vi "L_Cal_Data_Dis_Reflectivity.vi"(9 "Index(0 or 1)":i32, 10 "ID":i32, 11 "data":u8[](array[numeric])) -> (2 "reflectivity":u8, 3 "Distance":dbl)   [LabVIEW 2019]
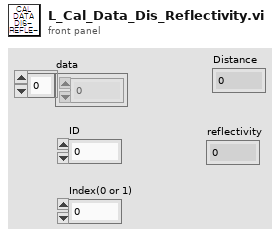
[diagram p1: front panel]
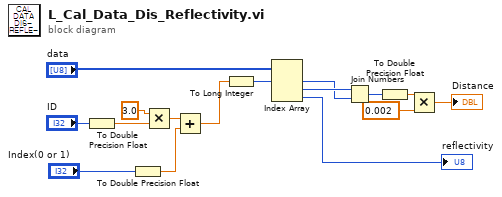
[diagram p0: block diagram]
diagram:
  n1 = To Double Precision Float(number="ID") -> (double precision float=w7:dbl)
  n2 = To Double Precision Float(number="Index(0 or 1)") -> (double precision float=w5:dbl)
  n3 = Multiply(x=3.0, y=w7) -> (x*y=w15:dbl)
  n4 = Add(x=w15, y=w5) -> (x+y=w3:dbl)
  n5 = To Long Integer(number=w3) -> (32bit integer=w4:i32)
  n6 = Index Array(array="data", index #1=w4) -> (element #1=w13:u8, element #2=w14:u8, element #3=→"reflectivity":u8)  [unwired: 2 in]
  n7 = Join Numbers(hi=w14, lo=w13) -> ((hi.lo)=w12:u16)
  n8 = To Double Precision Float(number=w12) -> (double precision float=w11:dbl)
  n9 = Multiply(x=w11, y=0.002) -> (x*y=→"Distance":dbl)
